vi "Do Something Else and Wait for Reply.vi"(6 "wait for reply (T)":bool=TRUE, 8 "error in (no error)":errorcluster, 9 "X":dbl, 10 "Do Something Message":string, 11 "TemplateAPI in":refnum<class "ExampleAPI.lvclass">) -> (0 "error out":errorcluster, 1 "timed out?":bool, 2 "Reply Payload":T1, 3 "TemplateAPI out":refnum<class "ExampleAPI.lvclass">)   [LabVIEW 2018, in "ExampleAPI.lvclass"]
uses:
  ExampleAPI.lvclass
  C:/Users/Phalanx/Documents/LabVIEW-Application-API-Template/src/Classes/AppControlAPI/AppControlAPI.lvclass
  Libraries/Example/Do Something Else and Wait (Reply Payload)--cluster.ctl
  AppControlAPI/AppControlAPI.lvclass/AppControlAPI.ctl
  4c94efee-2ba9-4b86-bf77-9303cd5a5534.vi
  AppControlAPI/Read AppRef.vi
  AppControlAPI/Insert In Reference Cache.vi
  AppControlAPI/Read Cache.vi
  AppControlAPI/Write Cache.vi
  Libraries/Example/Example.lvlib
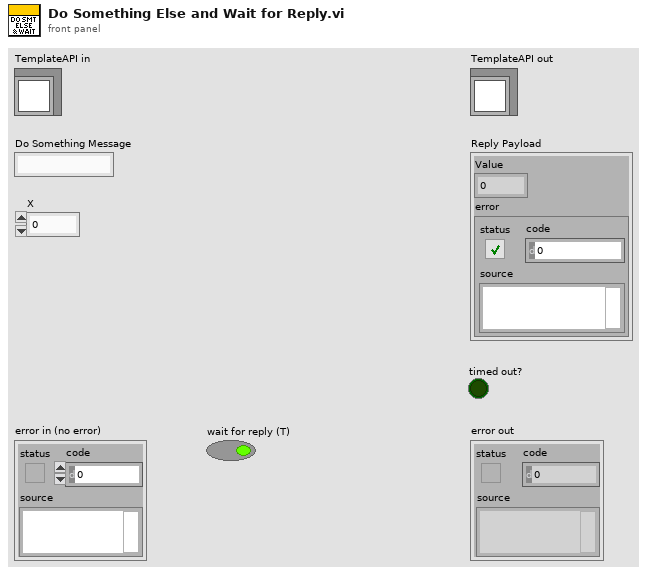
[diagram p1: front panel]
types:
  T1 = typedef "Example.lvlib/Do Something Else and Wait (Reply Payload)--cluster.ctl" = cluster{"Value":dbl, "error":errorcluster}
  T2 = typedef "Template.lvlib/Do Something Else and Wait (Reply Payload)--cluster.ctl" = cluster{"Value":dbl, "error":errorcluster}
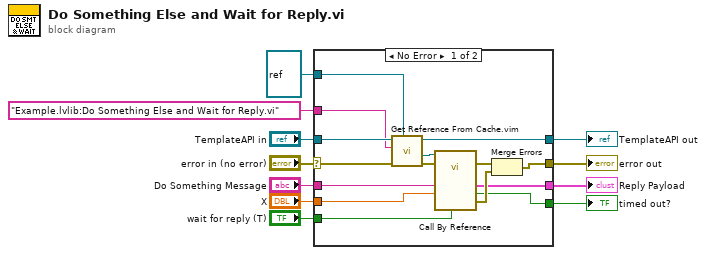
[diagram p0: block diagram]
diagram:
  n1 = case shown="No Error" "error in (no error)" {
    selector: "error in (no error)" -> [w22 w28]
    tunnel: [w19 w28] -> w10
    tunnel: [w25 w27] -> w8
    tunnel: "TemplateAPI in" -> [w26 w27]
    tunnel: "Do Something Message" -> [w20 _]
    tunnel: "Example.lvlib:Do Something Else and Wait for Reply.vi" ("VIQualifiedName") -> [w17 _]
    tunnel: refnum<vi> refnum ("type specifier VI Refnum (for type only)") -> [w16 _]
    tunnel: "X" -> [w15 _]
    tunnel: "wait for reply (T)" -> [w14 _]
    tunnel: [w13 _] -> w2
    tunnel: [w12 _] -> w1
    frame No Error {
      n2 = call "Get Reference From Cache.vim"("type specifier VI Refnum (for type only)"=w16, "error in (no error)"=w22, "VIQualifiedName"=w17, "AppControlAPI in"=w26) -> ("error out"=w23:errorcluster, "VIRef"=w24:refnum<vi>, "AppControlAPI out"=w25:refnum<class "ExampleAPI.lvclass">)  [unwired: 5 in]
      n3 = call-by-ref "?"(reference=w24, error in=w23, "wait for reply (T)"=w14, "X"=w15, "Do Something Else Message"=w20) -> (error out=w21:errorcluster, 0:"error out"=w18:errorcluster, "timed out?"=w12:bool, "Reply Payload"=w13:T2)  [unwired: 6 in, 1 out]
      n4 = Merge Errors(w21, w18) -> (w19:errorcluster)
    }
    frame Error {
    }
  }
  "error out" <- w10
  "TemplateAPI out" <- w8
  "Reply Payload" <- w2
  "timed out?" <- w1
